vi "Create Table.vi"() -> ()   [LabVIEW 2024]
uses:
  <vilib>/addons/database/Auxilliary.llb/DB Tools Column Info.ctl
  <vilib>/addons/database/Auxilliary.llb/DB Tools DataTypes.ctl
  <vilib>/addons/database/Connection.llb/DB Tools Open Connec (Path).vi
  <vilib>/addons/database/NI_Database_API.lvlib
panel:
  in  "column information":T1[](array[typedef])=[{"column name"="ID", "data type"=enum."String", "size"=10, "allow null?"=TRUE}, {"column name"="Grade", "data type"=enum."Long (I32)", "size"=10, "allow null?"=TRUE}]
  in  "connection information":path
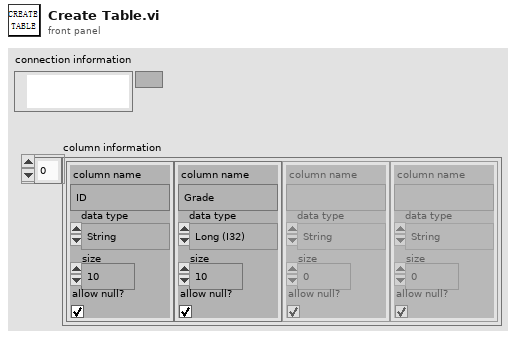
[diagram p1: front panel]
types:
  T1 = typedef "NI_Database_API.lvlib/DB Tools Column Info.ctl" = cluster{"column name":string, "data type":T2, "size":i32, "allow null?":bool}
  T2 = typedef "NI_Database_API.lvlib/DB Tools DataTypes.ctl" = enum16{"String", "Long (I32)", "Single (SGL)", "Double (DBL)", "Date/Time", "Binary"}
  T3 = typedef "NI_Database_API.lvlib/Conn ObjectReference.ctl" = refnum<k1>
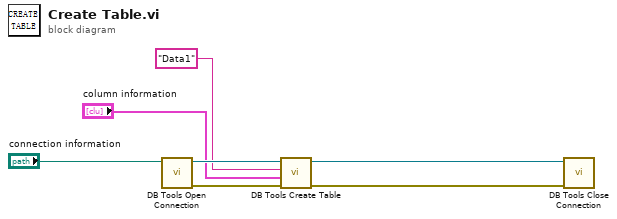
[diagram p0: block diagram]
diagram:
  n1 = call-poly <vilib>:"DB Tools Open Connection.vi"("connection information"="connection information") -> ("error out"=w4:errorcluster, "connection reference"=w7:T3)  [unwired: 7 in]
  n2 = call <vilib>:"DB Tools Create Table.vi"("error in (no error)"=w4, "column information"="column information", "table"="Data1", "connection reference"=w7) -> ("error out"=w5:errorcluster, "connection reference out"=w6:T3)  [unwired: 4 in]
  n3 = call <vilib>:"DB Tools Close Connection.vi"("error in (no error)"=w5, "connection reference"=w6) -> ()  [unwired: 5 in, 1 out]
